vi "Test Get Nonexisting Symbol.vi"(8 "error in (no error)":errorcluster, 11 "Test Case In":refnum<class "Conditional Disabled Configurator Test.lvclass">) -> (0 "error out":errorcluster, 3 "Test Case Out":refnum<class "Conditional Disabled Configurator Test.lvclass">)   [LabVIEW 2020, in "Conditional Disabled Configurator Test.lvclass"]
uses:
  Conditional Disabled Configurator Test.lvclass
  Conditional Disabled Configurator Test.lvclass/Conditional Disabled Configurator Test.ctl
  source/Conditional Disabled Configurator/Conditional Disabled Configurator.lvclass
  <vilib>/Astemes/LUnit/Test Case.lvclass
  C:/Program Files (x86)/National Instruments/LabVIEW 2020/vi.lib/Astemes/LUnit/Test Case.lvclass
  C:/Users/anton/Documents/GitHub/triarc-debugger/test/Conditional Disabled Configurator Test/Conditional Disabled Configurator Test.lvclass
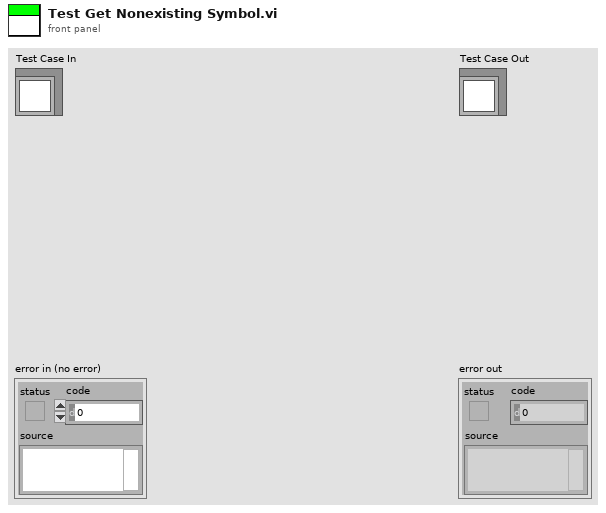
[diagram p1: front panel]
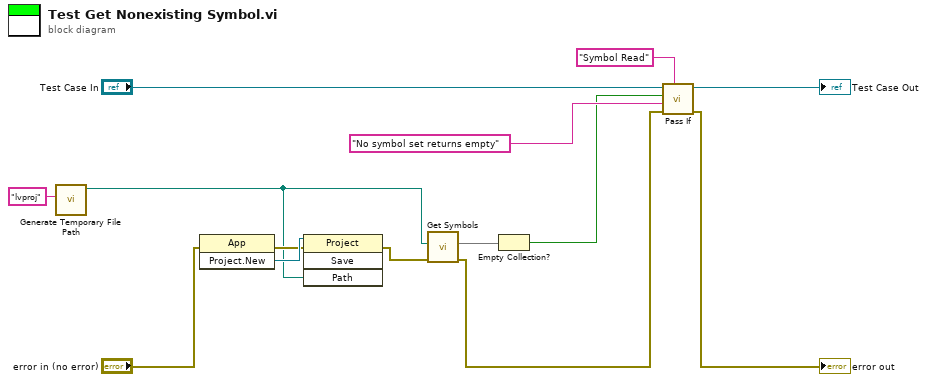
[diagram p0: block diagram]
diagram:
  n1 = call <vilib>:"Generate Temporary File Path.vi"("Temporary File Extension (tmp)"="lvproj") -> ("Unique Temporary File Path"=w5:path)  [unwired: 9 in, 1 out]
  n2 = invoke class="App" method="Project.New"(error in="error in (no error)") -> (error out=w6:errorcluster, "Project:New"=w7:refnum<vi>)  [unwired: 2 in, 1 out]
  n3 = invoke class="Project" method="Save"(reference=w7, error in=w6, "Path"=w5) -> (error out=w2:errorcluster)  [unwired: 1 in, 3 out]
  n4 = call "Get Symbols.vi"("error in (no error)"=w2, "Project Path"=w5) -> ("error out"=w11:errorcluster, "Symbols"=w4:map{string, string})  [unwired: 8 in]
  n5 = Empty Collection?(1:w4) -> (0:w3:bool)
  n6 = call <vilib>:"Pass If.vi"("Description"="Symbol Read", "error in (no error)"=w11, "Message"="No symbol set returns empty", "Pass?"=w3, "LUnit Test Case In"="Test Case In") -> ("error out"=→"error out":errorcluster, "LUnit Test Case Out"=→"Test Case Out":refnum<class "Conditional Disabled Configurator Test.lvclass">)  [unwired: 5 in]
